vi "GetValueTest.vi"() -> ()   [LabVIEW 2016]
uses:
  <vilib>/addons/_JKI Toolkits/Caraya/classes/Assert/Assert Equal Value and Type_Variant.vi
  <vilib>/addons/_JKI Toolkits/Caraya/classes/Assert/Assert.lvclass
  <vilib>/addons/_JKI Toolkits/Caraya/classes/Test/Test.lvclass
panel:
  out "error out":errorcluster
  in  "error in":errorcluster
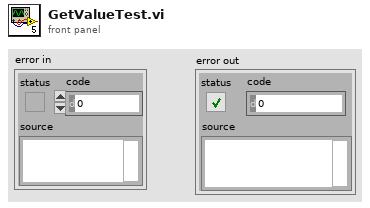
[diagram p1: front panel]
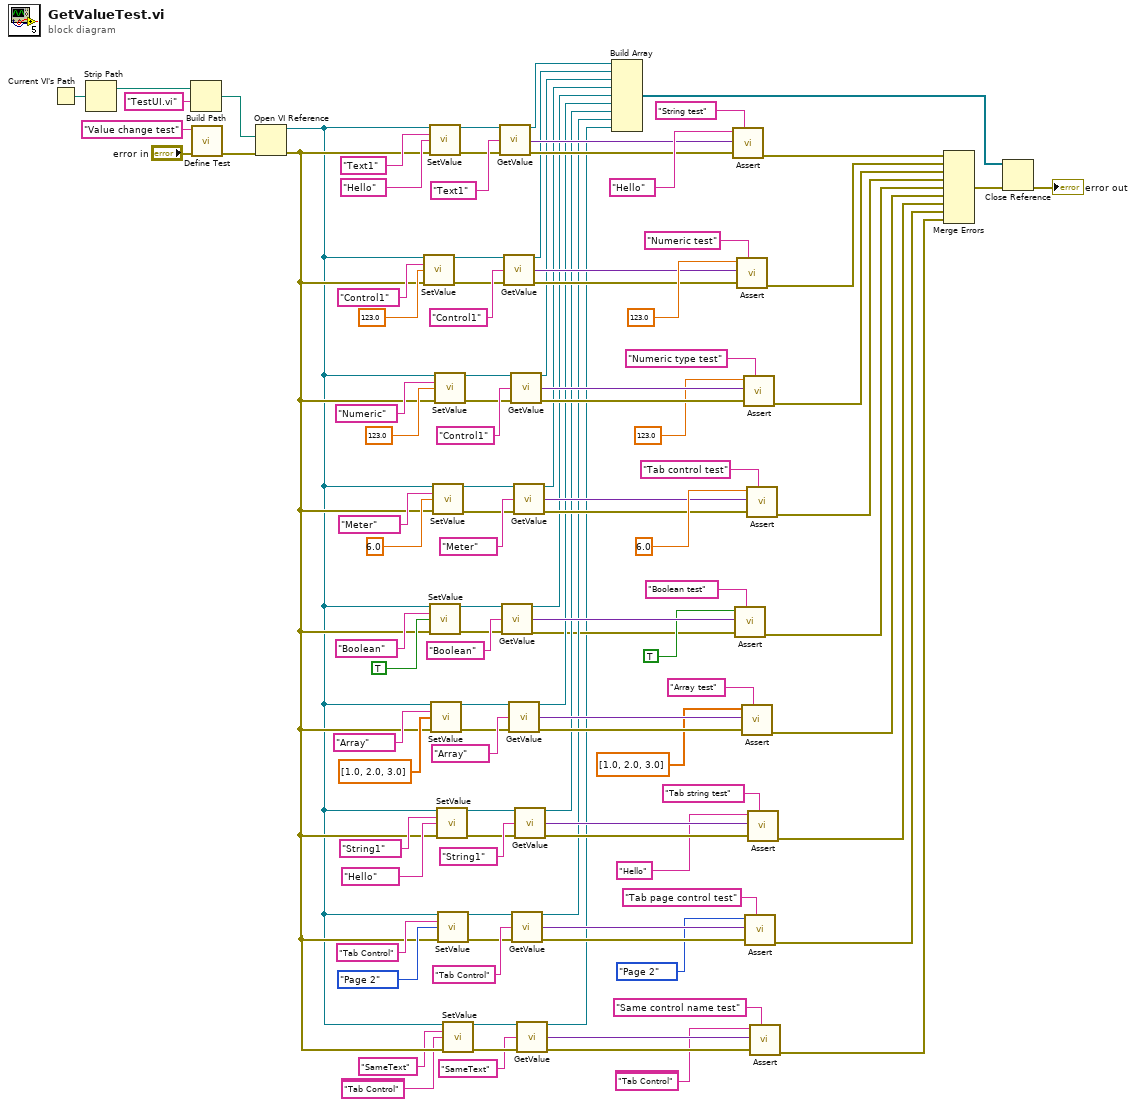
[diagram p0: block diagram]
diagram:
  (unwired) "Tab Control" ("Control Name")
  (unwired) "Tab Control" ("Control Name")
  n1 = Current VI's Path() -> (path=w5:path)
  n2 = Strip Path(path=w5) -> (stripped path=w4:path)  [unwired: 1 out]
  n3 = Build Path(base path=w4, name or relative path="TestUI.vi") -> (appended path=w3:path)
  n4 = call <vilib>:"Define Test.vi"("error in (no error)"="error in", "Label (VI Title)"="Value change test") -> ("error out"=w107:errorcluster)  [unwired: 9 in]
  n5 = Open VI Reference(vi path=w3, error in (no error)=w107) -> (vi reference=w1:refnum<vi>, error out=w12:errorcluster)  [unwired: 4 in]
  n6 = call "SetValue.vi"("VI Reference"=w1, "Control Name"="Control1", "Control Value"=123.0 ("Control Name"), "error in"=w12) -> ("VI Reference out"=w46:refnum<vi>, "error out"=w45:errorcluster)  [unwired: 10 in]
  n7 = call "SetValue.vi"("VI Reference"=w1, "Control Name"="Text1", "Control Value"="Hello" ("Control Name"), "error in"=w12) -> ("VI Reference out"=w50:refnum<vi>, "error out"=w48:errorcluster)  [unwired: 10 in]
  n8 = call "SetValue.vi"("VI Reference"=w1, "Control Name"="Boolean", "Control Value"=TRUE, "error in"=w12) -> ("VI Reference out"=w34:refnum<vi>, "error out"=w33:errorcluster)  [unwired: 10 in]
  n9 = call "SetValue.vi"("VI Reference"=w1, "Control Name"="Array", "Control Value"=dbl[] [1.0, 2.0, 3.0], "error in"=w12) -> ("VI Reference out"=w30:refnum<vi>, "error out"=w29:errorcluster)  [unwired: 10 in]
  n10 = call "SetValue.vi"("VI Reference"=w1, "Control Name"="Meter", "Control Value"=6.0 ("Control Name"), "error in"=w12) -> ("VI Reference out"=w38:refnum<vi>, "error out"=w37:errorcluster)  [unwired: 10 in]
  n11 = call "SetValue.vi"("VI Reference"=w1, "Control Name"="Numeric", "Control Value"=123.0 ("Control Name"), "error in"=w12) -> ("VI Reference out"=w42:refnum<vi>, "error out"=w41:errorcluster)  [unwired: 10 in]
  n12 = call "SetValue.vi"("VI Reference"=w1, "Control Name"="String1", "Control Value"="Hello" ("Control Name"), "error in"=w12) -> ("VI Reference out"=w26:refnum<vi>, "error out"=w25:errorcluster)  [unwired: 10 in]
  n13 = call "SetValue.vi"("VI Reference"=w1, "Control Name"="Tab Control", "Control Value"=enum32{"Page 1", "Page 2", "Page 3"}."Page 2" ("Tab Control"), "error in"=w12) -> ("VI Reference out"=w22:refnum<vi>, "error out"=w21:errorcluster)  [unwired: 10 in]
  n14 = call "SetValue.vi"("VI Reference"=w1, "Control Name"="SameText", "Control Value"="lol" ("Control Name"), "error in"=w12) -> ("VI Reference out"=w16:refnum<vi>, "error out"=w17:errorcluster)  [unwired: 10 in]
  n15 = call "GetValue.vi"("VI Reference"=w50, "Control Name"="Text1", "error in"=w48) -> ("VI Reference out"=w65:refnum<vi>, "Control Value"=w101:variant, "error out"=w102:errorcluster)  [unwired: 10 in]
  n16 = call "GetValue.vi"("VI Reference"=w34, "Control Name"="Boolean", "error in"=w33) -> ("VI Reference out"=w60:refnum<vi>, "Control Value"=w83:variant, "error out"=w52:errorcluster)  [unwired: 10 in]
  n17 = call "GetValue.vi"("VI Reference"=w46, "Control Name"="Control1", "error in"=w45) -> ("VI Reference out"=w63:refnum<vi>, "Control Value"=w99:variant, "error out"=w100:errorcluster)  [unwired: 10 in]
  n18 = call "GetValue.vi"("VI Reference"=w30, "Control Name"="Array", "error in"=w29) -> ("VI Reference out"=w59:refnum<vi>, "Control Value"=w78:variant, "error out"=w77:errorcluster)  [unwired: 10 in]
  n19 = call "GetValue.vi"("VI Reference"=w42, "Control Name"="Control1", "error in"=w41) -> ("VI Reference out"=w62:refnum<vi>, "Control Value"=w96:variant, "error out"=w95:errorcluster)  [unwired: 10 in]
  n20 = call "GetValue.vi"("VI Reference"=w22, "Control Name"="Tab Control", "error in"=w21) -> ("VI Reference out"=w53:refnum<vi>, "Control Value"=w56:variant, "error out"=w55:errorcluster)  [unwired: 10 in]
  n21 = call "GetValue.vi"("VI Reference"=w38, "Control Name"="Meter", "error in"=w37) -> ("VI Reference out"=w61:refnum<vi>, "Control Value"=w87:variant, "error out"=w88:errorcluster)  [unwired: 10 in]
  n22 = call "GetValue.vi"("VI Reference"=w26, "Control Name"="String1", "error in"=w25) -> ("VI Reference out"=w58:refnum<vi>, "Control Value"=w71:variant, "error out"=w72:errorcluster)  [unwired: 10 in]
  n23 = call "GetValue.vi"("VI Reference"=w16, "Control Name"="SameText", "error in"=w17) -> ("VI Reference out"=w11:refnum<vi>, "Control Value"=w14:variant, "error out"=w15:errorcluster)  [unwired: 10 in]
  n24 = Build Array(w65, w63, w62, w61, w60, w59, w58, w53, w11) -> (w64:refnum<vi>[])
  n25 = call-poly <vilib>:"Assert.vi"("Label"="String test", "error in (no error)"=w102, "Y"=w101, "X"="Hello" ("Control Name")) -> ("error out"=w98:errorcluster)  [unwired: 7 in]
  n26 = call-poly <vilib>:"Assert.vi"("Label"="Boolean test", "error in (no error)"=w52, "Y"=w83, "X"=TRUE) -> ("error out"=w81:errorcluster)  [unwired: 7 in]
  n27 = call-poly <vilib>:"Assert.vi"("Label"="Numeric test", "error in (no error)"=w100, "Y"=w99, "X"=123.0 ("Control Name")) -> ("error out"=w97:errorcluster)  [unwired: 7 in]
  n28 = call-poly <vilib>:"Assert.vi"("Label"="Array test", "error in (no error)"=w77, "Y"=w78, "X"=dbl[] [1.0, 2.0, 3.0]) -> ("error out"=w74:errorcluster)  [unwired: 7 in]
  n29 = call-poly <vilib>:"Assert.vi"("Label"="Numeric type test", "error in (no error)"=w95, "Y"=w96, "X"=123.0 ("Control Name")) -> ("error out"=w91:errorcluster)  [unwired: 7 in]
  n30 = call-poly <vilib>:"Assert.vi"("Label"="Tab page control test", "error in (no error)"=w55, "Y"=w56, "X"=enum32{"Page 1", "Page 2", "Page 3"}."Page 2" ("Tab Control")) -> ("error out"=w51:errorcluster)  [unwired: 7 in]
  n31 = call-poly <vilib>:"Assert.vi"("Label"="Tab control test", "error in (no error)"=w88, "Y"=w87, "X"=6.0 ("Control Name")) -> ("error out"=w85:errorcluster)  [unwired: 7 in]
  n32 = call-poly <vilib>:"Assert.vi"("Label"="Tab string test", "error in (no error)"=w72, "Y"=w71, "X"="Hello" ("Label")) -> ("error out"=w68:errorcluster)  [unwired: 7 in]
  n33 = call-poly <vilib>:"Assert.vi"("Label"="Same control name test", "error in (no error)"=w15, "Y"=w14, "X"="lol" ("Control Name")) -> ("error out"=w10:errorcluster)  [unwired: 7 in]
  n34 = Merge Errors(w98, w97, w91, w85, w81, w74, w68, w51, w10) -> (w67:errorcluster)
  n35 = Close Reference(reference=w64, error in (no error)=w67) -> (error out=→"error out":errorcluster)
